vi "Configure Synchronization Triggers.vi"(0 "TSM context":T1, 11 "error in (no error)":errorcluster) -> (15 "error out":errorcluster)   [LabVIEW 2020]
uses:
  <vilib>/NI_TestStand_SemiconductorModule/NI_TestStand_Semiconductor_Module.lvlibp/PinMap/General/SemiconductorModuleContext.ctl
  <vilib>/NI_TestStand_SemiconductorModule/NI_TestStand_Semiconductor_Module.lvlibp/PinMap/DAQmx/PinToNIDAQmxTask.vi
  <vilib>/NI_TestStand_SemiconductorModule/NI_TestStand_Semiconductor_Module.lvlibp/PinMap/DAQmx/PinToNIDAQmxTasks.vi
  <vilib>/NI_TestStand_SemiconductorModule/NI_TestStand_Semiconductor_Module.lvlibp
  <resource>/objmgr/daqmx.rc
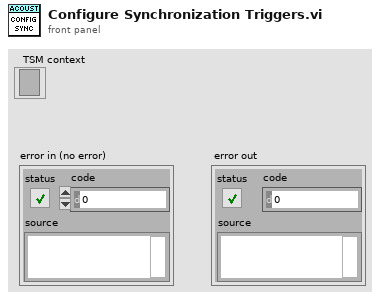
[diagram p1: front panel]
types:
  T1 = typedef "NI_TestStand_Semiconductor_Module.lvlibp/SemiconductorModuleContext.ctl" = refnum<k7>
  T2 = typedef "TSM DAQmx Multi-Task.ctl" = cluster{"Pin Query Context":refnum<class "MultiplePinMultipleSessionQueryContext.lvclass">, "SSC":T3[], "Site Numbers":i32[], "Pins":tag[]}
  T3 = typedef "SSC DAQmx.ctl" = cluster{"DAQmx Task ":refnum<k21>, "Channels":string, "Channel Lists":string}
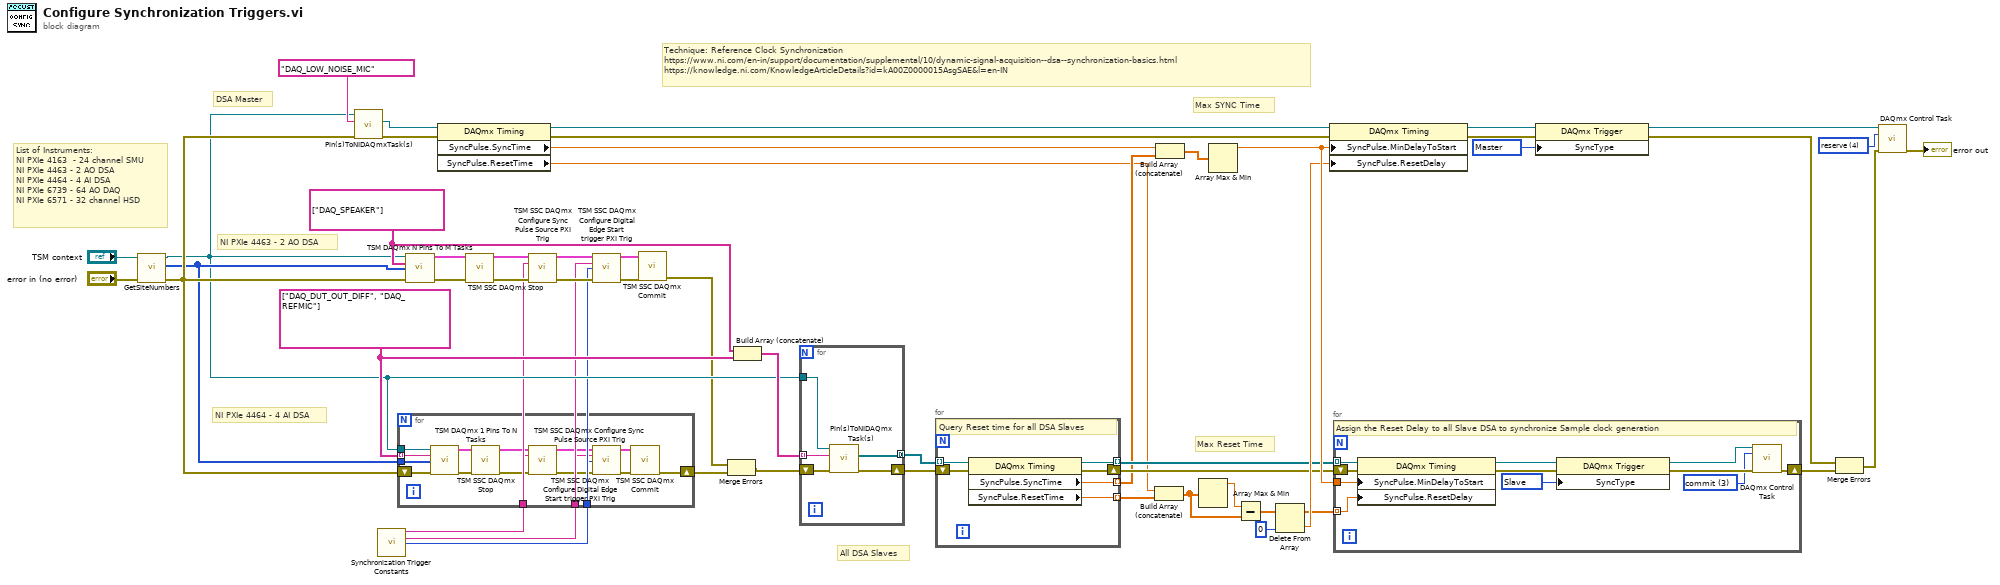
[diagram p0: block diagram]
diagram:
  w27 = 4 items=["verify"=2, "reserve"=4, "commit"=3, "unreserve"=5, "abort"=6] ("action")
  w25 = 15888 items=["None"=10230, "Master"=15888, "Slave"=15889] ("SyncType")
  w36 = tag[] ["DAQ_DUT_OUT_DIFF", "DAQ_REFMIC"] ("Pins")
  w37 = tag[] ["DAQ_SPEAKER"] ("Pins")
  # "Technique: Reference Clock Synchronization\nhttps://www.ni.com/en-in/support/documentation/supplemental/10/dynamic-signal-acquisition--dsa--synchronization-basics.html\nhttps://knowledge.ni.com/KnowledgeArticleDetails?id=kA00Z0000015AsgSAE&l=en-IN"
  # "Max Reset Time"
  # "Max SYNC Time"
  # "All DSA Slaves"
  # "DSA Master"
  # "NI PXIe 4464 - 4 AI DSA"
  # "NI PXIe 4463 - 2 AO DSA"
  # "List of Instruments:\nNI PXIe 4163  - 24 channel SMU\nNI PXIe 4463 - 2 AO DSA\nNI PXIe 4464 - 4 AI DSA\nNI PXIe 6739 - 64 AO DAQ\nNI PXIe 6571 - 32 channel HSD"
  n1 = call <vilib>:"GetSiteNumbers.vi"("error in (no error)"="error in (no error)", "Semiconductor Module Context"="TSM context") -> ("error out"=w41:errorcluster, "Site Numbers"=w40:i32[], "Semiconductor Module Context Out"=w34:T1)  [unwired: 6 in, 1 out]
  n2 = call-poly <vilib>:"Pin(s)ToNIDAQmxTask(s).vi"("error in (no error)"=w41, "Pin"=tag "DAQ_LOW_NOISE_MIC", "Semiconductor Module Context"=w34) -> ("error out"=w39:errorcluster, "DAQmx Task"=w38:refnum<k21>)  [unwired: 4 in, 3 out]
  n3 = call "Synchronization Trigger Constants.vi"() -> ("Sync Pulse"=w3:string, "Start Trigger"=w2:string, "Start Trigger Edge"=w1:i32)  [unwired: 13 in]
  n4 = for {
    tunnel: w40 -> [w59]
    tunnel: w36 -> [w58] mode=indexing
    tunnel: w34 -> [w57]
    tunnel: w3 -> [w55]
    tunnel: w2 -> [w54]
    tunnel: w1 -> [w53]
    shift-right: [w56] -> w33
    shift-left: w41 -> [w60]
    n5 = call "TSM DAQmx 1 Pins To N Tasks.vi"("TSM context"=w57, "Pins"=w58, "Site Numbers"=w59, "error in"=w60) -> ("DAQ TSM Out"=w65:T2, "error out"=w63:errorcluster)  [unwired: 10 in]
    n6 = call "TSM SSC DAQmx Stop.vi"("TSM DAQmx In"=w65, "error in (no error)"=w63) -> ("TSM DAQmx Out"=w66:T2, "error out"=w64:errorcluster)  [unwired: 12 in]
    n7 = call "TSM SSC DAQmx Configure Sync Pulse Source PXI Trig.vi"("DAQ TSM in"=w66, "source(PXI_Trig0)"=w55, "error in (no error)"=w64) -> ("DAQ TSM Out"=w61:T2, "error out"=w62:errorcluster)  [unwired: 11 in]
    n8 = call "TSM SSC DAQmx Configure Digital Edge Start trigger PXI Trig.vi"("DAQ TSM in"=w61, "source(PXI_Trig0)"=w54, "Edge"=w53, "error in (no error)"=w62) -> ("DAQ TSM Out"=w68:T2, "error out"=w67:errorcluster)  [unwired: 10 in]
    n9 = call "TSM SSC DAQmx Commit.vi"("TSM DAQmx In"=w68, "error in (no error)"=w67) -> ("error out"=w56:errorcluster)  [unwired: 12 in, 1 out]
  }
  n10 = call "TSM DAQmx N Pins To M Tasks.vi"("TSM context"=w34, "Pins"=w37, "Site Numbers"=w40, "error in"=w41) -> ("DAQ TSM Out"=w45:T2, "error out"=w47:errorcluster)  [unwired: 10 in]
  n11 = property class="DAQmx Timing"(reference=w38, error in=w39) -> (reference out=w11:refnum<k21>, error out=w12:errorcluster, "SyncPulse.SyncTime"=w8:dbl, "SyncPulse.ResetTime"=w6:dbl)
  n12 = call "TSM SSC DAQmx Stop.vi"("TSM DAQmx In"=w45, "error in (no error)"=w47) -> ("TSM DAQmx Out"=w44:T2, "error out"=w46:errorcluster)  [unwired: 12 in]
  n13 = call "TSM SSC DAQmx Configure Sync Pulse Source PXI Trig.vi"("DAQ TSM in"=w44, "source(PXI_Trig0)"=w3, "error in (no error)"=w46) -> ("DAQ TSM Out"=w49:T2, "error out"=w48:errorcluster)  [unwired: 11 in]
  n14 = call "TSM SSC DAQmx Configure Digital Edge Start trigger PXI Trig.vi"("DAQ TSM in"=w49, "source(PXI_Trig0)"=w2, "Edge"=w1, "error in (no error)"=w48) -> ("DAQ TSM Out"=w42:T2, "error out"=w43:errorcluster)  [unwired: 10 in]
  n15 = call "TSM SSC DAQmx Commit.vi"("TSM DAQmx In"=w42, "error in (no error)"=w43) -> ("error out"=w31:errorcluster)  [unwired: 12 in, 1 out]
  n16 = Merge Errors(w31, w33) -> (w32:errorcluster)
  n17 = Build Array (concatenate)(w37, w36) -> (w35:tag[])
  n18 = for {
    tunnel: w35 -> [w73] mode=indexing
    tunnel: w34 -> [w72]
    tunnel: [w69] -> w29 mode=concatenating
    shift-right: [w70] -> w30
    shift-left: w32 -> [w71]
    n19 = call-poly <vilib>:"Pin(s)ToNIDAQmxTask(s).vi"("error in (no error)"=w71, "Pin"=w73, "Semiconductor Module Context"=w72) -> ("error out"=w70:errorcluster, "DAQmx Tasks"=w69:refnum<k21>[])  [unwired: 4 in, 3 out]
  }
  n20 = for {
    tunnel: [w77] -> w9 mode=indexing
    shift-right: [w78] -> w10
    shift-left: w30 -> [w79]
    tunnel: w29 -> [w76] mode=indexing
    tunnel: [w75] -> w5 mode=indexing
    tunnel: [w74] -> w7 mode=indexing
    # "Query Reset time for all DSA Slaves"
    n21 = property class="DAQmx Timing"(reference=w76, error in=w79) -> (reference out=w77:refnum<k21>, error out=w78:errorcluster, "SyncPulse.SyncTime"=w74:dbl, "SyncPulse.ResetTime"=w75:dbl)
  }
  n22 = Build Array (concatenate)(w6, w5) -> (w22:dbl[])
  n23 = Build Array (concatenate)(w8, w7) -> (w24:dbl[])
  n24 = Array Max & Min(array=w22) -> (max value=w23:dbl)  [unwired: 3 out]
  n25 = Array Max & Min(array=w24) -> (max value=w19:dbl)  [unwired: 3 out]
  n26 = Subtract(x=w23, y=w22) -> (x-y=w18:dbl[])
  n27 = Delete From Array(array=w18, index=0) -> (deleted portion=w16:dbl, array with subset deleted=w15:dbl[])  [unwired: 1 in]
  n28 = property class="DAQmx Timing"(reference=w11, error in=w12, "SyncPulse.MinDelayToStart"=w19, "SyncPulse.ResetDelay"=w16) -> (reference out=w20:refnum<k21>, error out=w21:errorcluster)
  n29 = for {
    tunnel: w9 -> [w83] mode=indexing
    shift-right: [w85] -> w28
    shift-left: w10 -> [w89]
    tunnel: w19 -> [w81]
    tunnel: w15 -> [w80] mode=indexing
    w86 = 3 items=["verify"=2, "reserve"=4, "commit"=3, "unreserve"=5, "abort"=6] ("action")
    w90 = 15889 items=["None"=10230, "Master"=15888, "Slave"=15889] ("SyncType")
    # "Assign the Reset Delay to all Slave DSA to synchronize Sample clock generation"
    n30 = property class="DAQmx Timing"(reference=w83, error in=w89, "SyncPulse.MinDelayToStart"=w81, "SyncPulse.ResetDelay"=w80) -> (reference out=w82:refnum<k21>, error out=w84:errorcluster)
    n31 = property class="DAQmx Trigger"(reference=w82, error in=w84, "SyncType"=w90) -> (reference out=w88:refnum<k21>, error out=w87:errorcluster)
    n32 = call <vilib>:"DAQmx Control Task.vi"("task/channels in"=w88, "action"=w86, "error in"=w87) -> ("error out"=w85:errorcluster)  [unwired: 11 in, 1 out]
  }
  n33 = property class="DAQmx Trigger"(reference=w20, error in=w21, "SyncType"=w25) -> (reference out=w26:refnum<k21>, error out=w14:errorcluster)
  n34 = Merge Errors(w14, w28) -> (w13:errorcluster)
  n35 = call <vilib>:"DAQmx Control Task.vi"("task/channels in"=w26, "action"=w27, "error in"=w13) -> ("error out"=→"error out":errorcluster)  [unwired: 11 in, 1 out]
